vi "2-Single Sine Cycle.vi"() -> ()   [LabVIEW 2014]
panel:
  in  "Iterations":dbl
  out "Waveform Chart":dbl(graph)
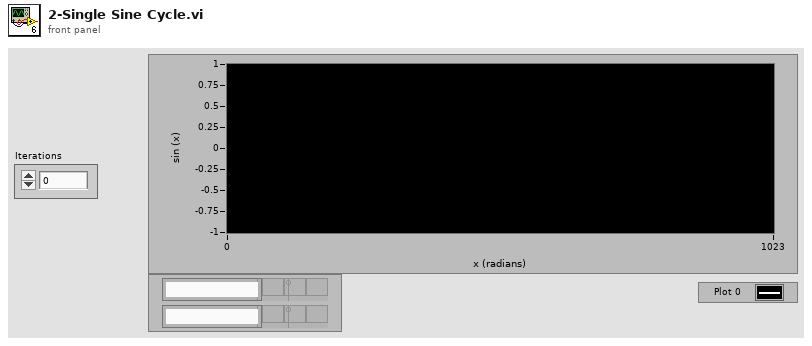
[diagram p1: front panel]
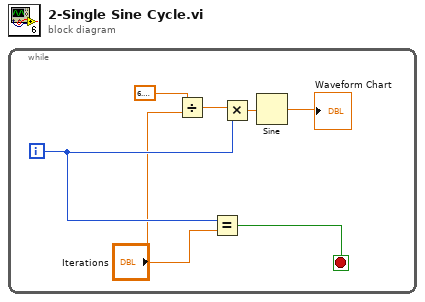
[diagram p0: block diagram]
diagram:
  n1 = while {
    i -> [w3]
    stop <- w7 stop-if-true
    n2 = Divide(x=6.283185307179586, y="Iterations") -> (x/y=w4:dbl)
    n3 = Equal?(x=w3, y="Iterations") -> (x = y?=w7:bool)
    n4 = Multiply(x=w4, y=w3) -> (x*y=w2:dbl)
    n5 = Sine(x=w2) -> (sin(x)=→"Waveform Chart":dbl)
  }
